vi "Save Log FGV.vi"(5 "Log Path":path=path "C:/Logs", 6 "Case":string, 7 "State":T1=enum."Init", 8 "Error In":errorcluster, 10 "Descripition":string, 11 "VI Name":string) -> (0 "Error Out":errorcluster)   [LabVIEW 2019, in "GUI.lvlib"]
uses:
  GUI.lvlib
  Controls/Save Log State.ctl
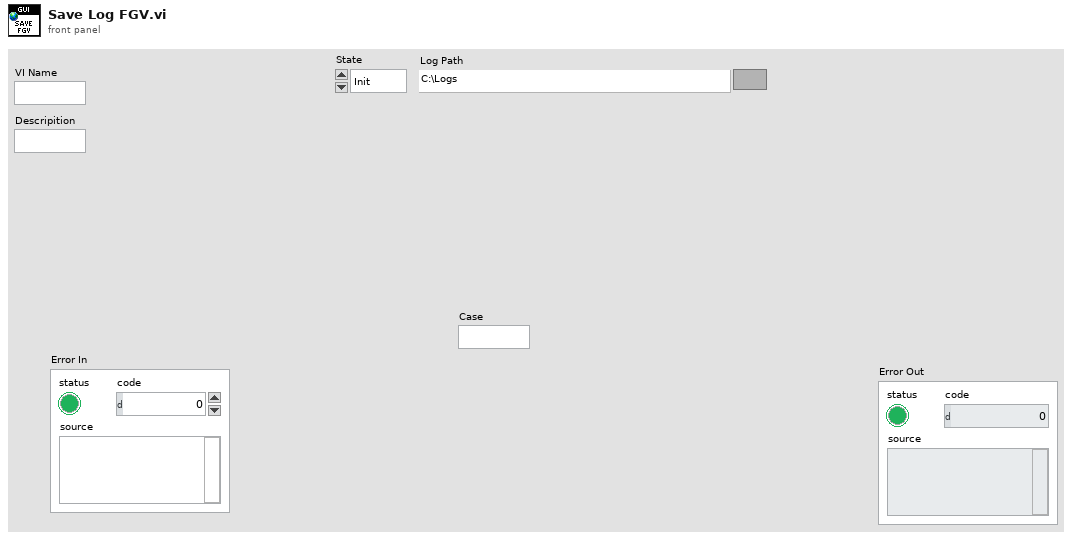
[diagram p1: front panel]
types:
  T1 = typedef "GUI.lvlib/Save Log State.ctl" = enum16{"Idle", "Init", "Write", "Exit"}
  T2 = enum16{"open", "replace", "create", "open or create", "replace or create", "replace or create with confirmation"}
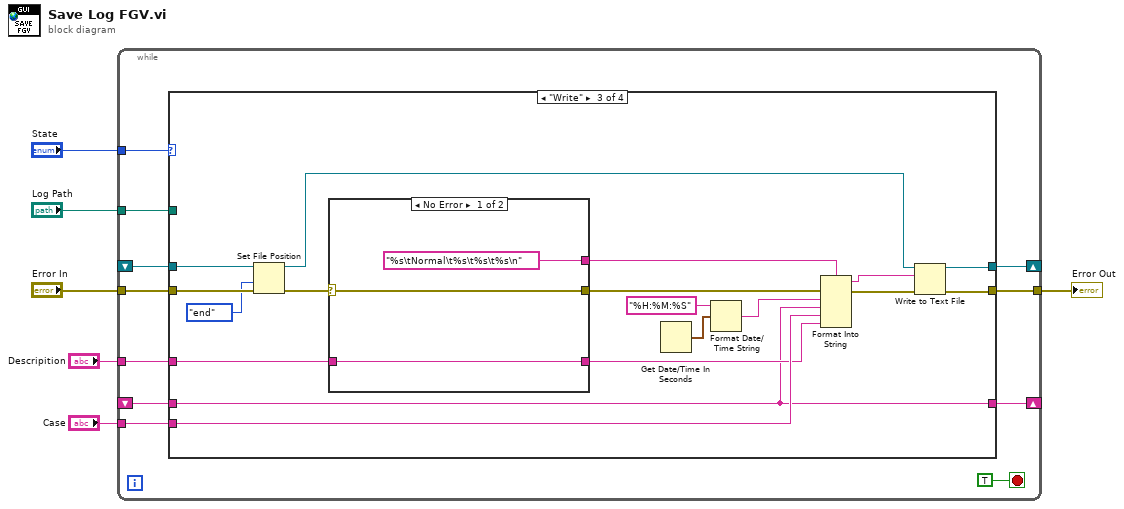
[diagram p0: block diagram]
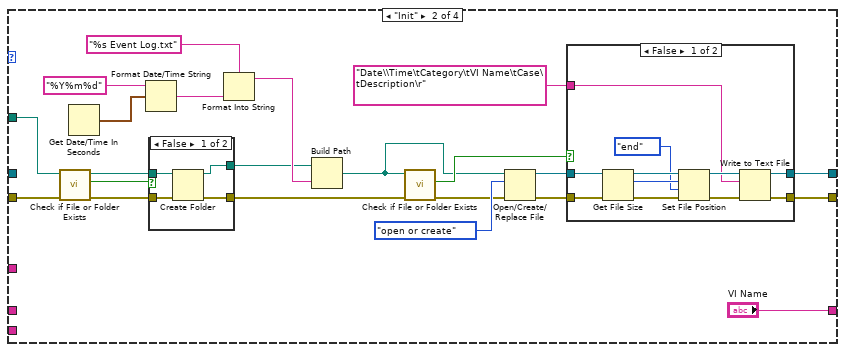
[diagram p3: hidden frame]
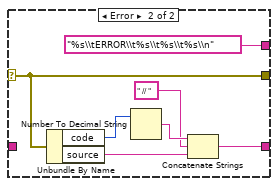
[diagram p6: hidden frame]
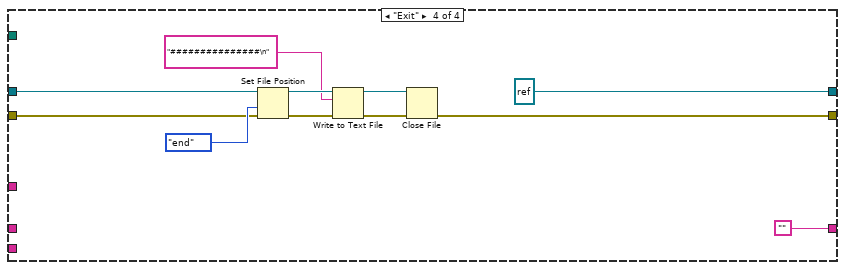
[diagram p7: hidden frame]
diagram:
  n1 = while {
    tunnel: "State" -> [w16]
    tunnel: "Error In" -> [w15]
    tunnel: [w14] -> w5
    tunnel: "Log Path" -> [w12]
    shift-right: [w13] -> _
    shift-left: _ -> [w11]
    tunnel: "Descripition" -> [w8]
    tunnel: "Case" -> [w7]
    shift-right: [w9] -> _
    shift-left: _ -> [w10]
    stop <- TRUE stop-if-true
    n2 = case shown="\"Write\"" w16 {
      tunnel: w15 -> [w19 w30 w79 w94]
      tunnel: [w19 w29 w76 w92] -> w14
      tunnel: [w20 w23 w75 refnum<file> refnum ("refnum out")] -> w13
      tunnel: w12 -> [_ w22 _ _]
      tunnel: w11 -> [w20 _ w77 w93]
      tunnel: w10 -> [w18 _ w63 _]
      tunnel: [w18 "VI Name" w63 ""] -> w9
      tunnel: w8 -> [_ _ w67 _]
      tunnel: w7 -> [_ _ w65 _]
      frame "Idle", Default {
      }
      frame "Init" {
        n3 = call <vilib>:"Check if File or Folder Exists.vi"("error in (no error)"=w30, "path"=w22) -> ("error out"=w28:errorcluster, "file or folder exists?"=w25:bool, "dup path"=w26:path)  [unwired: 7 in]
        n4 = Get Date/Time In Seconds() -> (seconds since 1Jan1904=w32:timestamp)
        n5 = Format Date/Time String(time format string (%c)="%Y%m%d", seconds (now)=w32) -> (date/time string=w33:string)  [unwired: 1 in]
        n6 = case shown="False" w25 {
          tunnel: w28 -> [w46 w48]
          tunnel: [w45 w48] -> w27
          tunnel: w26 -> [w44 w47]
          tunnel: [w43 w47] -> w24
          frame False {
            n7 = Create Folder(path (use dialog)=w44, error in=w46) -> (created path=w43:path, error out=w45:errorcluster)  [unwired: 1 in, 1 out]
          }
          frame True {
          }
        }
        n8 = Format Into String(format string="%s Event Log.txt" ("name or relative path"), w33) -> (resulting string=w34:string)  [unwired: 2 in, 1 out]
        n9 = Build Path(base path=w24, name or relative path=w34) -> (appended path=w36:path)
        n10 = call <vilib>:"Check if File or Folder Exists.vi"("error in (no error)"=w27, "path"=w36) -> ("error out"=w38:errorcluster, "file or folder exists?"=w37:bool)  [unwired: 7 in, 1 out]
        n11 = Open/Create/Replace File(file path (use dialog)=w36, error in=w38, operation (0:open)=T2."open or create") -> (refnum out=w35:refnum<file>, error out=w31:errorcluster)  [unwired: 3 in, 1 out]
        n12 = case shown="False" w37 {
          tunnel: w31 -> [w59 w60]
          tunnel: [w58 w60] -> w29
          tunnel: w35 -> [w55 w61]
          tunnel: [w57 w61] -> w23
          tunnel: "Date\\Time\tCategory\tVI Name\tCase\tDescription\r" ("text") -> [w50 _]
          frame False {
            n13 = Get File Size(file=w55, error in=w59) -> (refnum out=w53:refnum<file>, size (in bytes)=w51:i64, 0:w56:errorcluster)
            n14 = Set File Position(offset (in bytes) (0)=w51, refnum=w53, from (0:start)=enum16{"start", "end", "current"}."end", error in=w56) -> (refnum out=w52:refnum<file>, error out=w54:errorcluster)
            n15 = Write to Text File(file (use dialog)=w52, text=w50, error in=w54) -> (refnum out=w57:refnum<file>, error out=w58:errorcluster)  [unwired: 1 in, 1 out]
          }
          frame True {
          }
        }
      }
      frame "Write" {
        n16 = Set File Position(refnum=w77, from (0:start)=enum16{"start", "end", "current"}."end", error in=w79) -> (refnum out=w74:refnum<file>, error out=w78:errorcluster)  [unwired: 1 in]
        n17 = case shown="No Error" w78 {
          selector: w78 -> [w81 w83]
          tunnel: ["%s\tNormal\t%s\t%s\t%s\n" ("format string") "%s\\tERROR\\t%s\\t%s\\t%s\\n" ("format string")] -> w69
          tunnel: [w81 w83] -> w68
          tunnel: [w80 w84] -> w64
          tunnel: w67 -> [w80 _]
          frame No Error {
          }
          frame Error {
            n18 = Unbundle By Name(w83) -> ("code"=w89:i32, "source"=w87:string)
            n19 = Number To Decimal String(number=w89) -> (decimal integer string=w88:string)  [unwired: 1 in]
            n20 = Concatenate Strings(w88, " // ", w87) -> (w84:string)
          }
        }
        n21 = Get Date/Time In Seconds() -> (seconds since 1Jan1904=w72:timestamp)
        n22 = Format Date/Time String(time format string (%c)="%H:%M:%S", seconds (now)=w72) -> (date/time string=w66:string)  [unwired: 1 in]
        n23 = Format Into String(format string=w69, error in=w68, w66, w63, w65, w64) -> (resulting string=w62:string, error out=w70:errorcluster)  [unwired: 1 in]
        n24 = Write to Text File(file (use dialog)=w74, text=w62, error in=w70) -> (refnum out=w75:refnum<file>, error out=w76:errorcluster)  [unwired: 1 in, 1 out]
      }
      frame "Exit" {
        n25 = Set File Position(refnum=w93, from (0:start)=enum16{"start", "end", "current"}."end", error in=w94) -> (refnum out=w99:refnum<file>, error out=w98:errorcluster)  [unwired: 1 in]
        n26 = Write to Text File(file (use dialog)=w99, text="###############\n", error in=w98) -> (refnum out=w100:refnum<file>, error out=w96:errorcluster)  [unwired: 1 in, 1 out]
        n27 = Close File(refnum=w100, error in=w96) -> (error out=w92:errorcluster)  [unwired: 1 out]
      }
    }
  }
  "Error Out" <- w5
